vi "04.2 Invoke Node with Event-driven SM.vi"() -> ()   [LabVIEW 2019]
uses:
  Support Files/02.4 DAQmx Configuration Cluster.ctl
  Support Files/03.2 States.ctl
  Support Files/03.2 State Machine Data.ctl
  <vilib>/DAQmx/write.llb/DAQmx Write (Analog DBL 1Chan 1Samp).vi
  <vilib>/Utility/file.llb/Write Delimited Spreadsheet (string).vi
  <vilib>/Utility/file.llb/Write Delimited Spreadsheet (DBL).vi
  <vilib>/DAQmx/create/channels.llb/DAQmx Create Channel (AO-Voltage-Basic).vi
  <vilib>/DAQmx/miscellaneous.llb/DAQmx Fill In Error Info.vi
panel:
  in  "DAQmx Configuration Cluster":T1={"Desired Sample Rate (Hz)"=-1.0, "sample mode"=10178, "Minimum value"=-1.0, "Maximum value"=-1.0, "Physical Channel"="", "units"=10143, "thermocouple type"=10072, "Samples per Channel"=0} {"thermocouple type" items=["J"=10072, "K"=10073, "N"=10077, "R"=10082, "S"=10085, "T"=10086, "B"=10047, "E"=10055]; "units" items=["Deg C"=10143, "Deg F"=10144, "Kelvins"=10325, "Deg R"=10145, "From Custom Scale"=10065]; "sample mode" items=["Finite Samples"=10178, "Continuous Samples"=10123, "Hardware Timed Single Point"=12522]}
  in  "Threshold (RMS)":dbl
  in  "Generate Stimulus":bool
  in  "Stop":bool
  in  "Clear":bool
  in  "Acquire":bool
  out "Graph":dbl[][](graph)
  out "Thershold Exceeded?":bool
  out "RMS Result per Channel":dbl[](array[numeric])
  # "ANALYSIS"
  # "EVENTS"
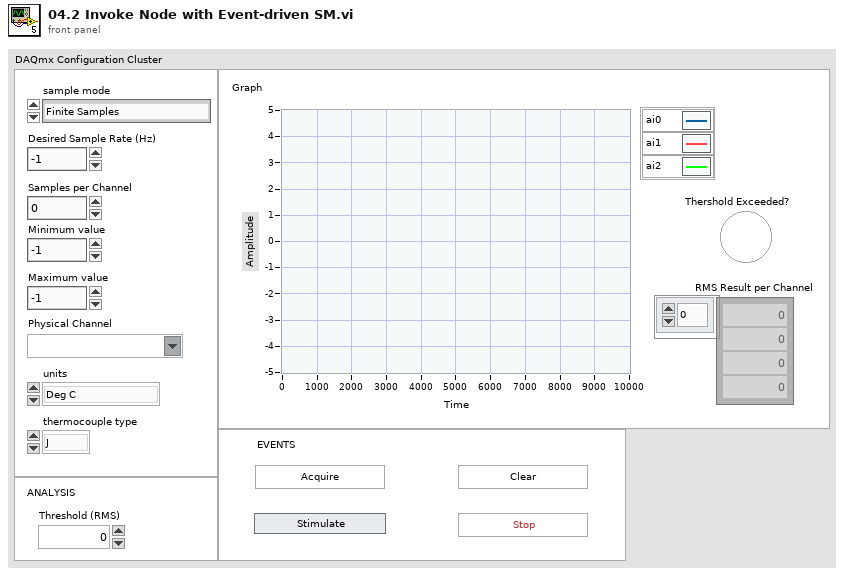
[diagram p1: front panel]
types:
  T1 = typedef "02.4 DAQmx Configuration Cluster.ctl" = cluster{"Desired Sample Rate (Hz)":dbl, "sample mode":i32, "Minimum value":dbl, "Maximum value":dbl, "Physical Channel":tag, "units":i32, "thermocouple type":i32, "Samples per Channel":i32}
  T2 = enum16{"Always On", "Always Off", "Off While Running"}
  T3 = typedef "03.2 State Machine Data.ctl" = cluster{"Acquisition Data":dbl[][], "Stimulus?":bool}
  T4 = typedef "03.2 States.ctl" = enum16{"Initialize", "Update UI", "Update Stimulus", "Wait for event", "Acquire", "Analyze", "Log", "Clear", "Shutdown"}
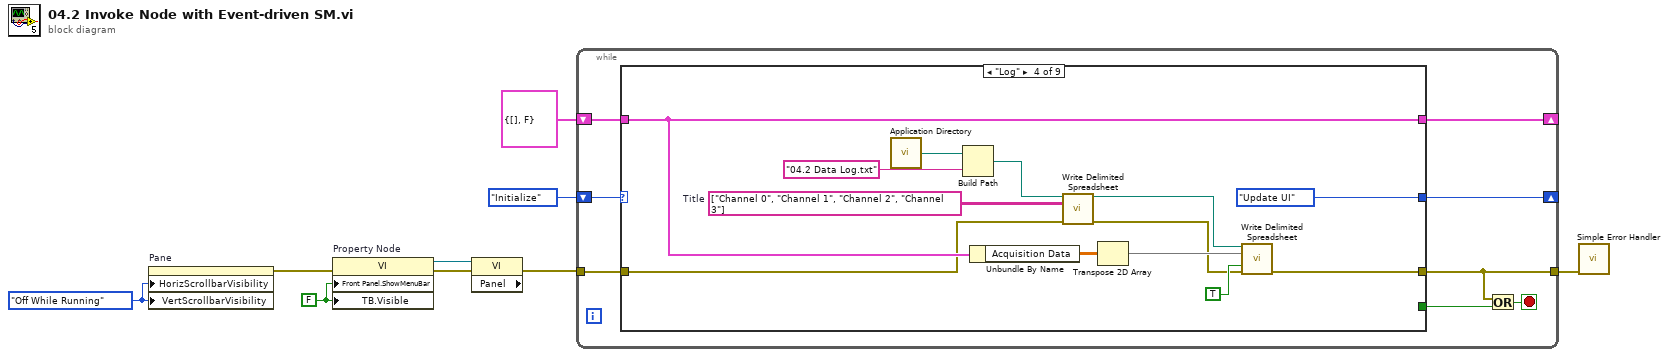
[diagram p0: block diagram]
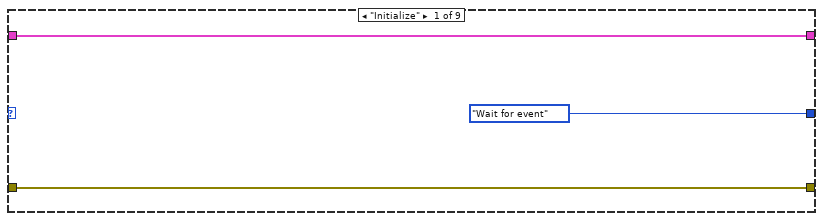
[diagram p2: hidden frame]
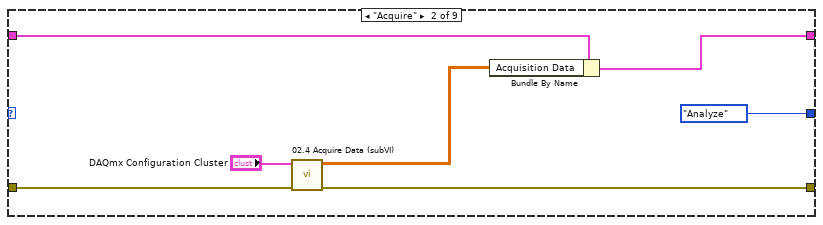
[diagram p3: hidden frame]
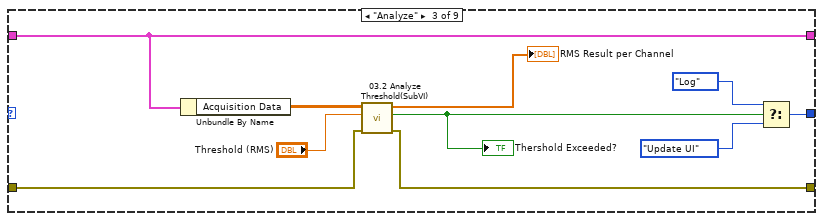
[diagram p4: hidden frame]
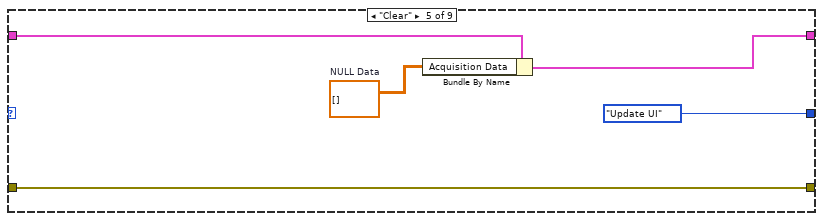
[diagram p5: hidden frame]
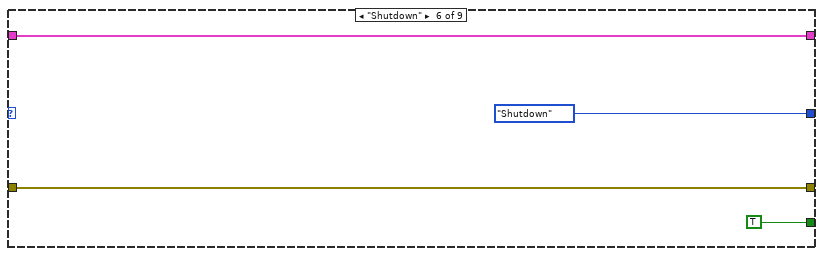
[diagram p6: hidden frame]
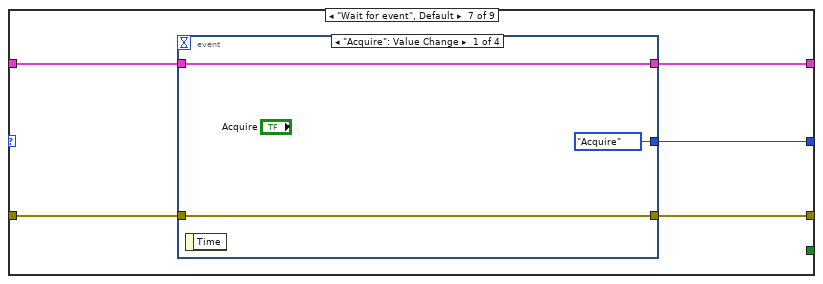
[diagram p7: hidden frame]
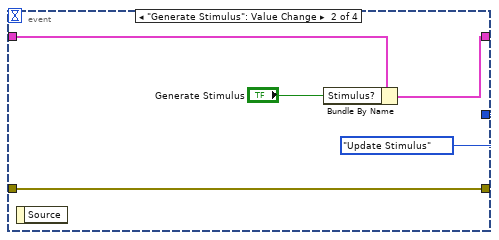
[diagram p8: hidden frame]
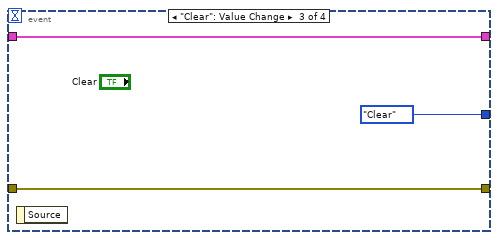
[diagram p9: hidden frame]
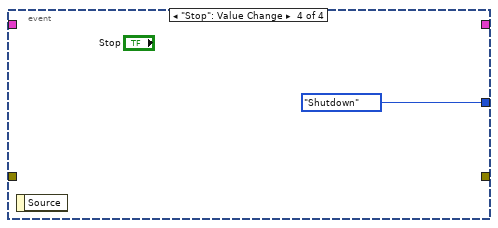
[diagram p10: hidden frame]
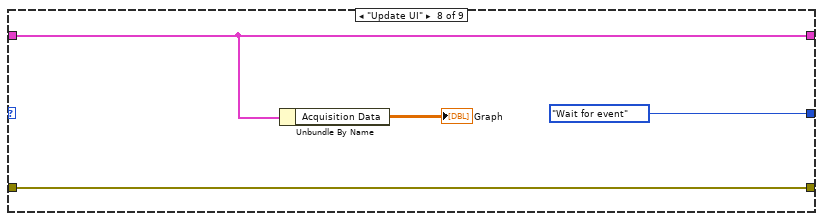
[diagram p11: hidden frame]
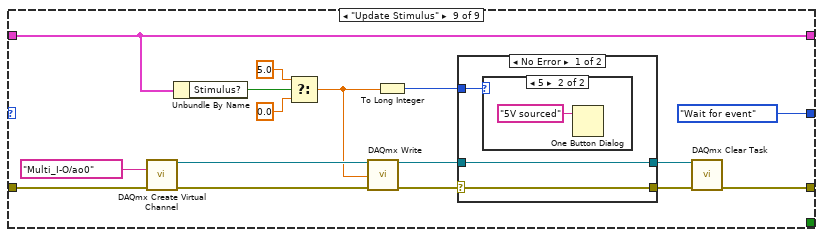
[diagram p12: hidden frame]
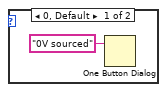
[diagram p13: hidden frame]
diagram:
  w5 = FALSE ("Tool Bar:Visible")
  w6 = T2."Off While Running" ("Horizontal Scrollbar Visibility")
  n1 = property on="Pane" class="Pane"("HorizScrollbarVisibility"=w6, "VertScrollbarVisibility"=w6) -> (error out=w4:errorcluster)  [unwired: 2 in, 1 out]
  n2 = property on="Property Node" class="VI"(error in=w4, "Front Panel.ShowMenuBar"=w5, "TB.Visible"=w5) -> (reference out=w3:refnum<vi>, error out=w2:errorcluster)  [unwired: 1 in]
  n3 = property class="VI" props=["Panel"](reference=w3, error in=w2) -> (error out=w1:errorcluster)  [unwired: 2 out]
  n4 = while {
    shift-right: [w16] -> _
    shift-left: 03.2_States."Initialize" ("State") -> [w17]
    tunnel: w1 -> [w15]
    tunnel: [w13] -> w8
    shift-right: [w12] -> _
    shift-left: T3 {"Acquisition Data"=[], "Stimulus?"=FALSE} -> [w11]
    stop <- w14 stop-if-true
    n5 = case shown="\"Log\"" w17 {
      tunnel: [03.2_States."Wait for event" ("State") 03.2_States."Analyze" ("State") w36 03.2_States."Update UI" ("State") 03.2_States."Update UI" ("State") 03.2_States."Shutdown" ("State") w64 03.2_States."Wait for event" ("State") 03.2_States."Wait for event" ("State")] -> w16
      tunnel: [w19 w23 w31 w48 w51 w57 w63 w78 w85] -> w13
      tunnel: w15 -> [w19 w24 w32 w38 w51 w57 w62 w78 w96]
      tunnel: [w20 w26 w30 w46 w54 w58 w61 w80 w82] -> w12
      tunnel: w11 -> [w20 w27 w30 w46 w55 w58 w60 w80 w82]
      tunnel: [_ _ _ _ _ TRUE _ _ _] -> w10
      frame "Initialize" {
      }
      frame "Acquire" {
        n6 = call "02.4 Acquire Data (subVI).vi"("Error In"=w24, "DAQmx Configuration Cluster"="DAQmx Configuration Cluster") -> ("error out"=w23:errorcluster, "2D DBL"=w25:dbl[][])  [unwired: 8 in]
        n7 = Bundle By Name(cluster=w27, "Acquisition Data"=w25) -> (w26:T3)
      }
      frame "Analyze" {
        n8 = Unbundle By Name(w30) -> ("Acquisition Data"=w37:dbl[][])
        n9 = call "03.2 Analyze Threshold(SubVI).vi"("Error In"=w32, "Threshold (RMS)"="Threshold (RMS)", "Data"=w37) -> ("Error Out"=w31:errorcluster, "Threshold exceeded?"=w33:bool, "RMS Results per Channel"=→"RMS Result per Channel":dbl[])  [unwired: 6 in]
        "Thershold Exceeded?" <- w33
        n10 = Select(t=03.2_States."Log" ("State"), s=w33, f=03.2_States."Update UI" ("State")) -> (s? t:f=w36:T4)
      }
      frame "Log" {
        w40 = string[][] [["Channel 0", "Channel 1", "Channel 2", "Channel 3"]]  # Title
        n11 = call <vilib>:"Application Directory.vi"() -> ("Application Directory"=w50:path)
        n12 = Build Path(base path=w50, name or relative path="04.2 Data Log.txt") -> (appended path=w41:path)
        n13 = Unbundle By Name(w46) -> ("Acquisition Data"=w45:dbl[][])
        n14 = call-poly <vilib>:"Write Delimited Spreadsheet.vi"("file path (dialog if empty)"=w41, "2D data"=w40, "error in (no error)"=w38) -> ("new file path (Not A Path if cancelled)"=w43:path, "error out"=w39:errorcluster)  [unwired: 11 in]
        n15 = Transpose 2D Array(2D array=w45) -> (transposed array=w44:dbl[][])
        n16 = call-poly <vilib>:"Write Delimited Spreadsheet.vi"("file path (dialog if empty)"=w43, "2D data"=w44, "append to file? (new file:F)"=TRUE, "error in (no error)"=w39) -> ("error out"=w48:errorcluster)  [unwired: 10 in, 1 out]
      }
      frame "Clear" {
        w53 = dbl[][] []  # NULL Data
        n17 = Bundle By Name(cluster=w55, "Acquisition Data"=w53) -> (w54:T3)
      }
      frame "Shutdown" {
      }
      frame "Wait for event", Default {
        n18 = event shown="[0] \"Acquire\": Value Change" {
          selector: _ -> [_ _ _ _]
          dyn-events: _ -> [_ _ _ _]
          timeout: _ -> [_ _ _ _]
          tunnel: [03.2_States."Acquire" ("State") 03.2_States."Update Stimulus" ("State") 03.2_States."Clear" ("State") 03.2_States."Shutdown" ("State")] -> w64
          tunnel: [w66 w68 w73 _] -> w63
          tunnel: w62 -> [w66 w68 w73 _]
          tunnel: [w65 w70 w75 _] -> w61
          tunnel: w60 -> [w65 w72 w75 _]
          event "Acquire": Value Change {
            n19 = event-data() -> ()  [unwired: 1 in, 1 out]
          }
          event "Generate Stimulus": Value Change {
            n20 = event-data() -> ()  [unwired: 1 in, 1 out]
            n21 = Bundle By Name(cluster=w72, "Stimulus?"="Generate Stimulus") -> (w70:T3)
          }
          event "Clear": Value Change {
            n22 = event-data() -> ()  [unwired: 1 in, 1 out]
          }
          event "Stop": Value Change {
            n23 = event-data() -> ()  [unwired: 1 in, 1 out]
          }
        }
      }
      frame "Update UI" {
        n24 = Unbundle By Name(w80) -> ("Acquisition Data"=→"Graph":dbl[][])
      }
      frame "Update Stimulus" {
        n25 = call-poly <vilib>:"DAQmx Create Virtual Channel.vi"("physical channels"=tag "Multi_I-O/ao0", "error in"=w96) -> ("task out"=w94:refnum<k21>, "error out"=w95:errorcluster)  [unwired: 12 in]
        n26 = Unbundle By Name(w82) -> ("Stimulus?"=w93:bool)
        n27 = Select(t=5.0, s=w93, f=0.0) -> (s? t:f=w90:dbl)
        n28 = call-poly <vilib>:"DAQmx Write.vi"("task/channels in"=w94, "data"=w90, "error in"=w95) -> ("task out"=w88:refnum<k21>, "error out"=w89:errorcluster)  [unwired: 10 in, 1 out]
        n29 = To Long Integer(number=w90) -> (32bit integer=w83:i32)
        n30 = case shown="No Error" w89 {
          selector: w89 -> [w99 w102]
          tunnel: w88 -> [w98 w103]
          tunnel: [w99 w102] -> w87
          tunnel: [w98 w103] -> w86
          tunnel: w83 -> [w97 _]
          frame No Error {
            n31 = case shown="5" w97 {
              frame 0, Default {
                n32 = One Button Dialog(message="0V sourced") -> ()  [unwired: 1 in, 1 out]
              }
              frame 5 {
                n33 = One Button Dialog(message="5V sourced") -> ()  [unwired: 1 in, 1 out]
              }
            }
          }
          frame Error {
          }
        }
        n34 = call <vilib>:"DAQmx Clear Task.vi"("task in"=w86, "error in"=w87) -> ("error out"=w85:errorcluster)  [unwired: 13 in]
      }
    }
    n35 = Or(x=w13, y=w10) -> (x .or. y?=w14:bool)
  }
  n36 = call <vilib>:"Simple Error Handler.vi"("error in (no error)"=w8) -> ()  [unwired: 4 in, 5 out]
